vi "Thermocouple.vi"() -> ()   [LabVIEW 2009]
uses:
  <vilib>/DAQmx/configure/timing.llb/DAQmx Timing (Sample Clock).vi
  <vilib>/DAQmx/create/channels.llb/DAQmx Create Channel (AI-Temperature-Thermocouple).vi
  <vilib>/DAQmx/read.llb/DAQmx Read (Analog DBL 1Chan 1Samp).vi
  Program Files/National Instruments/LabVIEW 2009/resource/objmgr/daqmx.rc
panel:
  in  "Sample Rate":dbl=1.0 format="%0.2f"
  in  "cjc source":i32(ring)=10200 items=["Built-In"=10200, "Constant Value"=10116, "Channel"=10113]
  in  "minimum value (degrees)":dbl=15.0 format="%0.2f"
  in  "maximum value (degrees)":dbl=35.0 format="%0.2f"
  in  "units":i32(ring)=10143 items=["Deg C"=10143, "Deg F"=10144, "Kelvins"=10325, "Deg R"=10145, "From Custom Scale"=10065]
  out "Thermocouple Data":cluster{"Temperature Limit":dbl, "data":dbl}(graph)
  out "Limit Exceeded?":bool
  in  "Temperature Limit":dbl(slide)=30.0 scale=20.0..35.0
  in  "stop":bool
  in  "Thermocouple Type":i32(ring)=10072 items=["J"=10072, "K"=10073, "N"=10077, "R"=10082, "S"=10085, "T"=10086, "B"=10047, "E"=10055]
  in  "Thermocouple Channel":tag="cDAQ1Mod1/ai1"
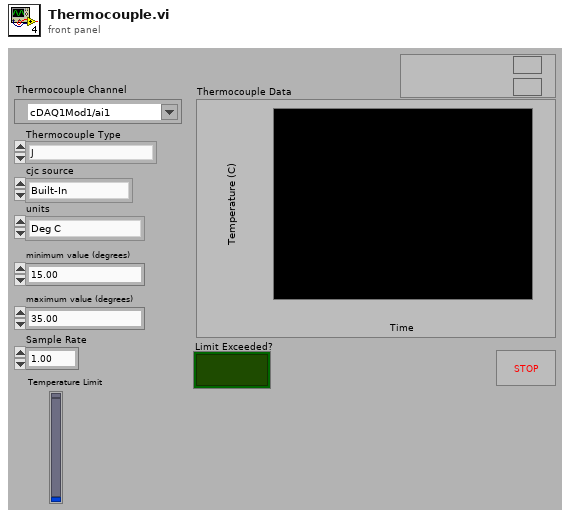
[diagram p1: front panel]
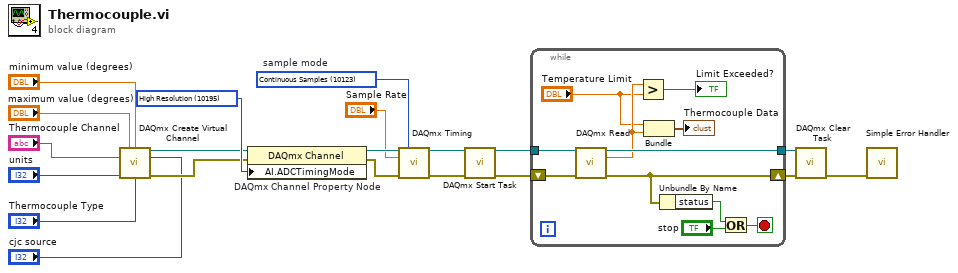
[diagram p0: block diagram]
diagram:
  w2 = 10123 items=["Finite Samples"=10178, "Continuous Samples"=10123, "Hardware Timed Single Point"=12522]  # sample mode
  w10 = 10195 items=["High Resolution"=10195, "High Speed"=14712, "Best 50 Hz Rejection"=14713, "Best 60 Hz Rejection"=14714] ("AI.ADCTimingMode")
  n1 = call-poly <vilib>:"DAQmx Create Virtual Channel.vi"("maximum value"="maximum value (degrees)", "minimum value"="minimum value (degrees)", "physical channels"="Thermocouple Channel", "cjc source"="cjc source", "units"="units", "thermocouple type"="Thermocouple Type") -> ("task out"=w9:refnum<k21>, "error out"=w8:errorcluster)  [unwired: 8 in]
  n2 = property on="DAQmx Channel Property Node" class="DAQmx Channel"(reference=w9, error in=w8, "AI.ADCTimingMode"=w10) -> (reference out=w6:refnum<k21>, error out=w4:errorcluster)
  n3 = call-poly <vilib>:"DAQmx Timing.vi"("task/channels in"=w6, "sample mode"=w2, "rate"="Sample Rate", "error in"=w4) -> ("task out"=w5:refnum<k21>, "error out"=w3:errorcluster)  [unwired: 10 in]
  n4 = call <vilib>:"DAQmx Start Task.vi"("task/channels in"=w5, "error in"=w3) -> ("task out"=w18:refnum<k21>, "error out"=w17:errorcluster)  [unwired: 12 in]
  n5 = while {
    tunnel: [w31] -> w14
    tunnel: w18 -> [w29]
    shift-right: [w28] -> w20
    shift-left: w17 -> [w30]
    stop <- w27 stop-if-true
    n6 = call-poly <vilib>:"DAQmx Read.vi"("task/channels in"=w29, "error in"=w30) -> ("task out"=w31:refnum<k21>, "data"=w24:dbl, "error out"=w28:errorcluster)  [unwired: 11 in]
    n7 = Greater?(x=w24, y="Temperature Limit") -> (0:→"Limit Exceeded?":bool)
    n8 = Bundle "Bundle"("Temperature Limit"="Temperature Limit", "data"=w24) -> (→"Thermocouple Data":cluster{"Temperature Limit":dbl, "data":dbl})  [unwired: 1 in]
    n9 = Unbundle By Name "Unbundle By Name"(w28) -> ("status"=w26:bool)
    n10 = Or(x=w26, y="stop") -> (x .or. y?=w27:bool)
  }
  n11 = call <vilib>:"DAQmx Clear Task.vi"("task in"=w14, "error in"=w20) -> ("error out"=w19:errorcluster)  [unwired: 13 in]
  n12 = call <vilib>:"Simple Error Handler.vi"("error in (no error)"=w19) -> ()  [unwired: 4 in, 5 out]
